vi "GetDescription.vi"(8 "error in (no error)":errorcluster, 11 "TestSuite in":refnum<class "TestSuite.lvclass">) -> (0 "error out":errorcluster, 2 "Description":string, 3 "TestSuite out":refnum<class "TestSuite.lvclass">)   [LabVIEW 2013, in "TestSuite.lvclass"]
uses:
  TestSuite.lvclass
  <userlib>/_OpenG.lib/string/string.llb/Trim Whitespace (String)__ogtk.vi
  Libraries/VITesterUtilities.lvlib
panel:
  # "JKI VI Tester for LabVIEW\nhttp://jkisoft.com/vi-tester\nCopyright (C) 2007-2009, JKI <info@jkisoft.com>\nALL RIGHTS RESERVED"
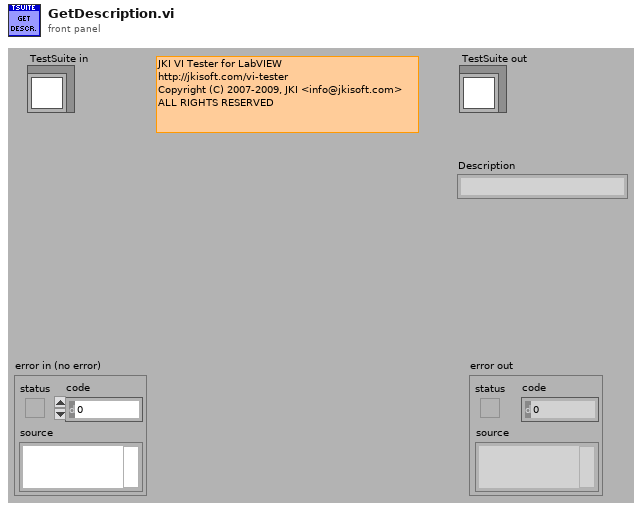
[diagram p1: front panel]
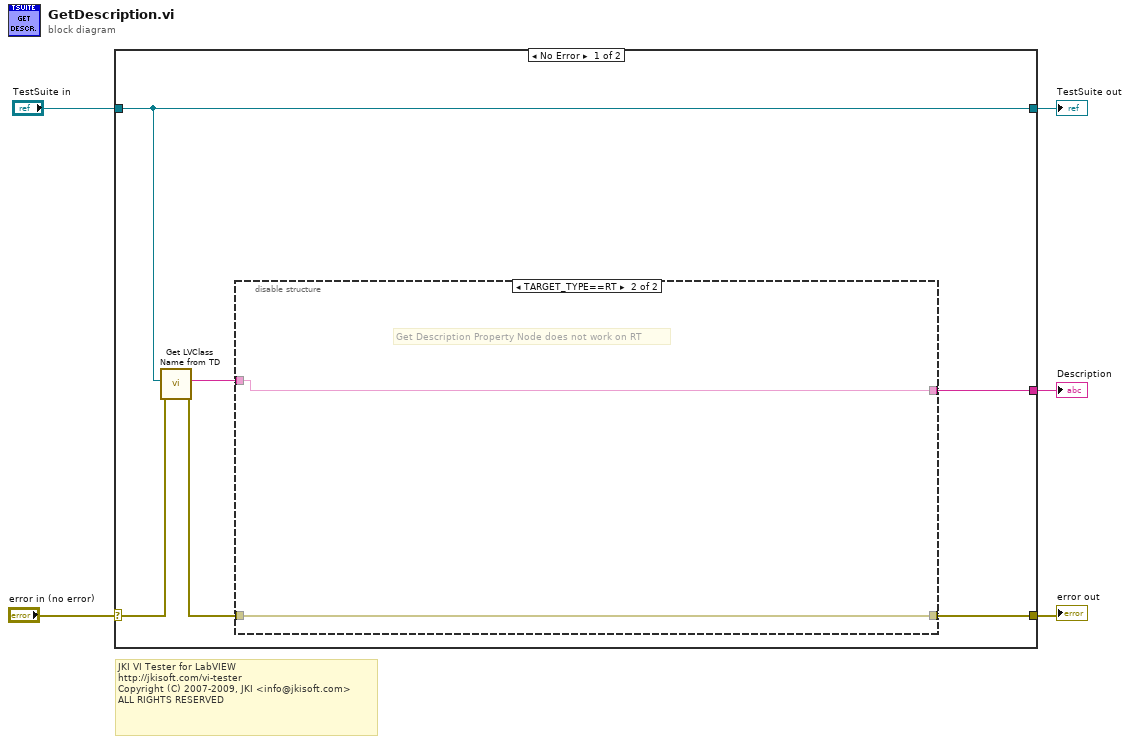
[diagram p0: block diagram]
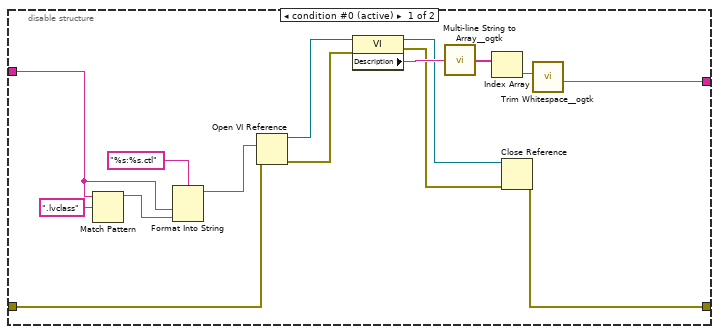
[diagram p2: hidden frame]
diagram:
  # "JKI VI Tester for LabVIEW\nhttp://jkisoft.com/vi-tester\nCopyright (C) 2007-2009, JKI <info@jkisoft.com>\nALL RIGHTS RESERVED"
  n1 = case shown="No Error" "error in (no error)" {
    selector: "error in (no error)" -> [w10 w30]
    tunnel: [w7 w30] -> w4
    tunnel: [w11 w29] -> w2
    tunnel: "TestSuite in" -> [w11 w29]
    tunnel: [w9 _] -> w1
    frame No Error {
      n2 = call "Get LVClass Name from TD.vi"("error in"=w10, "Variant"=w11) -> ("error out"=w8:errorcluster, "LVClass Name"=w6:string)  [unwired: 8 in]
      n3 = disable-structure shown="TARGET_TYPE==RT" {
        disable-tunnel: [w22 w28] -> w9
        disable-tunnel: w8 -> [w18 w27]
        disable-tunnel: [w17 w27] -> w7
        disable-tunnel: w6 -> [w12 w28]
        frame condition #0 (active) {
          n4 = Match Pattern(string=w12, regular expression=".lvclass") -> (before substring=w14:string)  [unwired: 1 in, 3 out]
          n5 = Format Into String(format string="%s:%s.ctl", w12, w14) -> (resulting string=w13:string)  [unwired: 2 in, 1 out]
          n6 = Open VI Reference(vi path=w13, error in (no error)=w18) -> (vi reference=w23:refnum<vi>, error out=w20:errorcluster)  [unwired: 4 in]
          n7 = property class="VI"(reference=w23, error in=w20) -> (reference out=w21:refnum<vi>, error out=w19:errorcluster, "Description"=w26:string)
          n8 = call <userlib>:"Multi-line String to Array__ogtk.vi"("string"=w26) -> ("lines"=w25:string[])
          n9 = Index Array(array=w25) -> (element=w24:string)  [unwired: 1 in]
          n10 = Close Reference(reference=w21, error in (no error)=w19) -> (error out=w17:errorcluster)
          n11 = call-poly <userlib>:"Trim Whitespace__ogtk.vi"("String in"=w24) -> ("String out"=w22:string)  [unwired: 6 in]
        }
        frame condition #1 {
          # "Get Description Property Node does not work on RT"
        }
      }
    }
    frame Error {
    }
  }
  "error out" <- w4
  "TestSuite out" <- w2
  "Description" <- w1
